vi "Example.vi"() -> ()   [LabVIEW 2025]
uses:
  libzmq-v143-mt-4_3_6/LibZMQ.lvlib
  libzmq-v143-mt-4_3_6/ctls/SocketType.ctl
panel:
  out "buf out":string
  out "Present":bool
  in  "TCP":bool
  out "error out 5":errorcluster
  out "error out 4":errorcluster
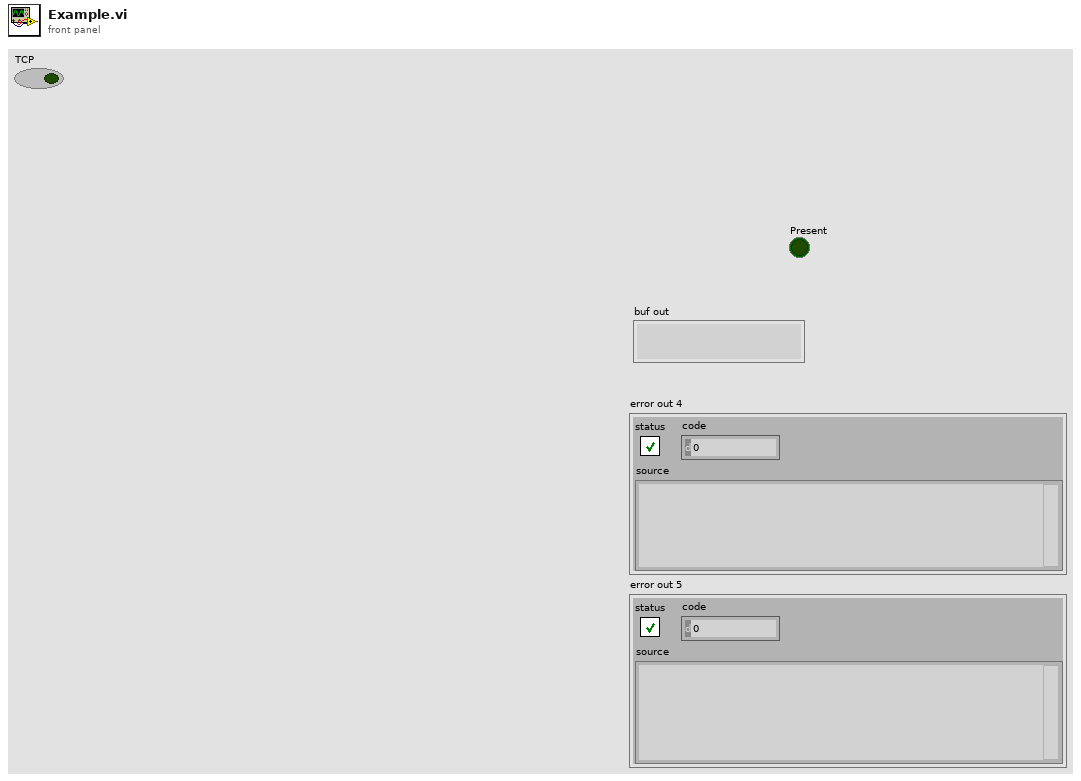
[diagram p1: front panel]
types:
  T1 = typedef "LibZMQ.lvlib/SocketType.ctl" = enum16{"Pair", "Pub", "Sub", "Request", "Reply", "Dealer", "Router", "Pull", "Push", "XPub", "XSub"}
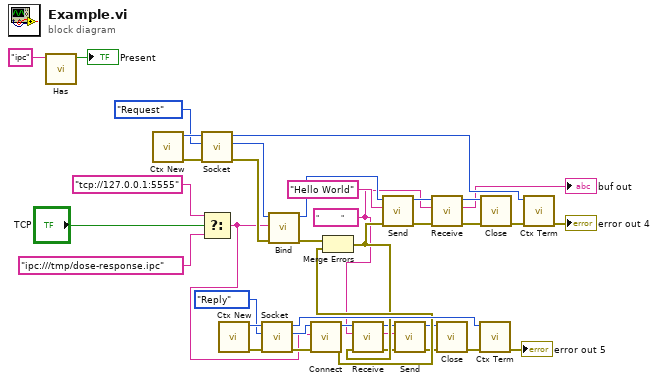
[diagram p0: block diagram]
diagram:
  w6 = "           " ("buf")
  n1 = call "Has.vi"("capability_"="ipc") -> ("Has"=→"Present":bool)  [unwired: 9 in, 1 out]
  n2 = call "Ctx New.vi"() -> ("error out"=w34:errorcluster, "function return"=w36:u64)  [unwired: 10 in]
  n3 = call "Socket.vi"("error in (no error)"=w34, "Socket Type"=SocketType."Request", "ctx in"=w36) -> ("error out"=w32:errorcluster, "s_"=w33:u64, "ctx out"=w35:u64)  [unwired: 6 in]
  n4 = Select(t="tcp://127.0.0.1:5555", s="TCP", f="ipc:///tmp/dose-response.ipc") -> (s? t:f=w15:string)
  n5 = call "Ctx New.vi"() -> ("error out"=w29:errorcluster, "function return"=w28:u64)  [unwired: 10 in]
  n6 = call "Socket.vi"("error in (no error)"=w29, "Socket Type"=SocketType."Reply", "ctx in"=w28) -> ("error out"=w27:errorcluster, "s_"=w26:u64, "ctx out"=w24:u64)  [unwired: 6 in]
  n7 = call "Bind.vi"("error in (no error)"=w32, "addr_"=w15, "s_"=w33) -> ("error out"=w30:errorcluster, "s_ out"=w31:u64)  [unwired: 7 in]
  n8 = call "Connect.vi"("error in (no error)"=w27, "addr_"=w15, "s_"=w26) -> ("error out"=w21:errorcluster, "s_ out"=w23:u64)  [unwired: 7 in]
  n9 = Merge Errors(w30, w21) -> (w20:errorcluster)
  n10 = call "Receive.vi"("error in (no error)"=w20, "buf in"=w6, "s"=w23) -> ("error out"=w2:errorcluster, "buf out"=w9:string, "s_"=w11:u64)  [unwired: 6 in]
  n11 = call "Send.vi"("error in (no error)"=w20, "buf"="Hello World", "s"=w31) -> ("error out"=w7:errorcluster, "s_"=w8:u64)  [unwired: 7 in]
  n12 = call "Send.vi"("error in (no error)"=w2, "buf"=w9, "s"=w11) -> ("error out"=w1:errorcluster, "s_"=w10:u64)  [unwired: 7 in]
  n13 = call "Receive.vi"("error in (no error)"=w7, "buf in"=w6, "s"=w8) -> ("error out"=w5:errorcluster, "buf out"=→"buf out":string, "s_"=w4:u64)  [unwired: 6 in]
  n14 = call "Close.vi"("error in (no error)"=w1, "s_"=w10) -> ("error out"=w25:errorcluster)  [unwired: 9 in]
  n15 = call "Ctx Term.vi"("error in (no error)"=w25, "context_"=w24) -> ("error out"=→"error out 5":errorcluster)  [unwired: 9 in]
  n16 = call "Close.vi"("error in (no error)"=w5, "s_"=w4) -> ("error out"=w37:errorcluster)  [unwired: 9 in]
  n17 = call "Ctx Term.vi"("error in (no error)"=w37, "context_"=w35) -> ("error out"=→"error out 4":errorcluster)  [unwired: 9 in]
